vi "Control Limelight.vi"(0 "Read Data Loop Time (ms) (min 10)":u32, 2 "Write Data Loop Time (ms)":u32) -> ()   [LabVIEW 2018]
uses:
  <vilib>/Rock Robotics/Network Tables/NT Read Number.vi
  Robot Global Data.vi
  <vilib>/Rock Robotics/Network Tables/NT Write Number.vi
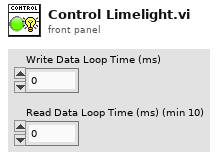
[diagram p1: front panel]
types:
  T1 = cluster{"offsetAngle H":dbl, "offsetAngle V":dbl, "area":dbl, "skew":dbl, "validTarget":dbl, "latency":dbl}
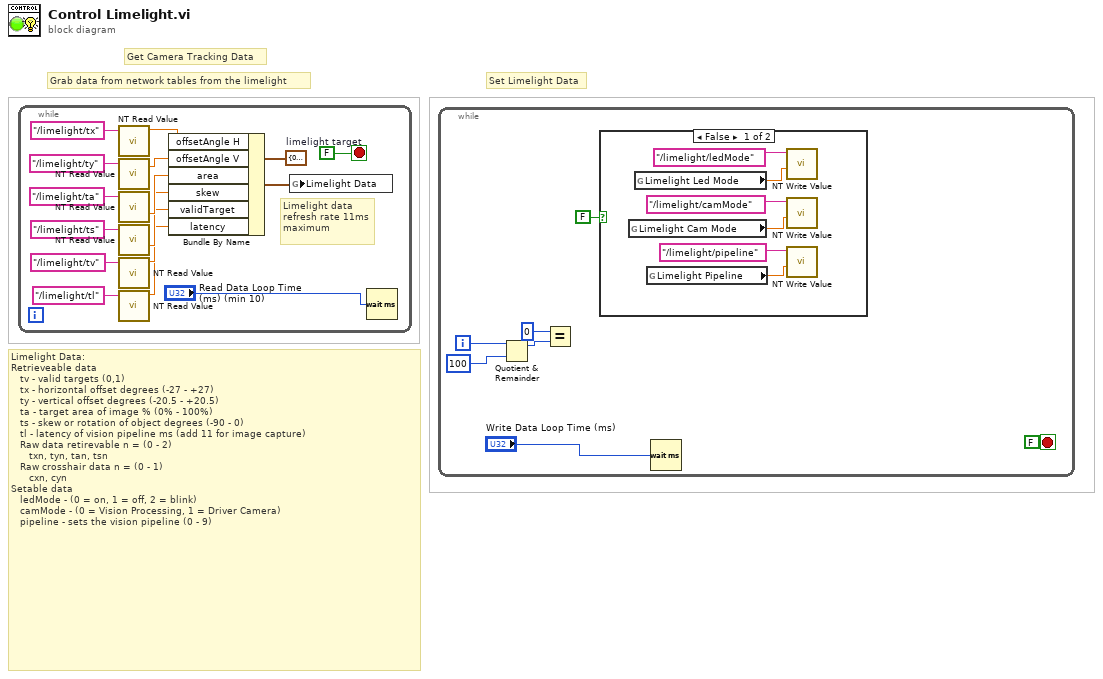
[diagram p0: block diagram]
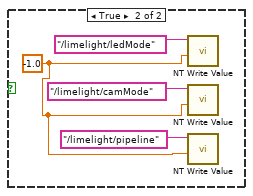
[diagram p2: hidden frame]
diagram:
  # "Set Limelight Data"
  # "Limelight Data:\nRetrieveable data\n   tv - valid targets (0,1)\n   tx - horizontal offset degrees (-27 - +27)\n   ty - vertical offset degrees (-20.5 - +20.5)\n   ta - target area of image % (0% - 100%)\n   ts - skew or rotation of object degrees (-90 - 0)\n   tl - latency of vision pipeline ms (add 11 for image capture)\n   Raw data retirevable n = (0 - 2)\n      txn, tyn, tan, tsn\n   Raw crosshair data n = (0 - 1)\n      cxn, cyn\nSetable data\n   ledMode - (0 = on, 1 = off, 2 = blink)\n   camMode - (0 = Vision Processing, 1 = Driver Camera)\n   pipeline - sets the vision pipeline (0 - 9)"
  # "Grab data from network tables from the limelight"
  # "Get Camera Tracking Data"
  n1 = while {
    stop <- FALSE stop-if-true
    w12 = T1 {"offsetAngle H"=0.0, "offsetAngle V"=0.0, "area"=0.0, "skew"=0.0, "validTarget"=0.0, "latency"=0.0}  # limelight target
    # "Limelight data\nrefresh rate 11ms\nmaximum"
    n2 = call-poly <vilib>:"NT Read Value.vi"("Name"="/limelight/tx") -> ("Numeric"=w11:dbl)  [unwired: 9 in, 1 out]
    n3 = call-poly <vilib>:"NT Read Value.vi"("Name"="/limelight/ty") -> ("Numeric"=w10:dbl)  [unwired: 9 in, 1 out]
    n4 = call-poly <vilib>:"NT Read Value.vi"("Name"="/limelight/ta") -> ("Numeric"=w9:dbl)  [unwired: 9 in, 1 out]
    n5 = call-poly <vilib>:"NT Read Value.vi"("Name"="/limelight/ts") -> ("Numeric"=w8:dbl)  [unwired: 9 in, 1 out]
    n6 = call-poly <vilib>:"NT Read Value.vi"("Name"="/limelight/tv") -> ("Numeric"=w4:dbl)  [unwired: 9 in, 1 out]
    n7 = call-poly <vilib>:"NT Read Value.vi"("Name"="/limelight/tl") -> ("Numeric"=w2:dbl)  [unwired: 9 in, 1 out]
    n8 = Bundle By Name(cluster=w12, "offsetAngle H"=w11, "offsetAngle V"=w10, "area"=w9, "skew"=w8, "validTarget"=w4, "latency"=w2) -> (w6:T1)
    n9 = global write "Robot Global Data.vi" "Limelight Data"(w6) -> ()
    n10 = Wait (ms)(milliseconds to wait="Read Data Loop Time (ms) (min 10)") -> ()  [unwired: 1 out]
  }
  n11 = while {
    i -> [w21]
    stop <- FALSE stop-if-true
    n12 = Quotient & Remainder(x=w21, y=100) -> (x-y*floor(x/y)=w19:i32)  [unwired: 1 out]
    n13 = Equal?(x=0, y=w19) -> ()  [unwired: 1 out]
    n14 = case shown="False" FALSE {
      frame False {
        n15 = global read "Robot Global Data.vi" "Limelight Cam Mode"() -> (w25:dbl)
        n16 = global read "Robot Global Data.vi" "Limelight Led Mode"() -> (w26:dbl)
        n17 = global read "Robot Global Data.vi" "Limelight Pipeline"() -> (w24:dbl)
        n18 = call-poly <vilib>:"NT Write Value.vi"("Numeric"=w26, "Name"="/limelight/ledMode") -> ()  [unwired: 9 in, 1 out]
        n19 = call-poly <vilib>:"NT Write Value.vi"("Numeric"=w25, "Name"="/limelight/camMode") -> ()  [unwired: 9 in, 1 out]
        n20 = call-poly <vilib>:"NT Write Value.vi"("Numeric"=w24, "Name"="/limelight/pipeline") -> ()  [unwired: 9 in, 1 out]
      }
      frame True {
        w30 = -1.0
        n21 = call-poly <vilib>:"NT Write Value.vi"("Numeric"=w30, "Name"="/limelight/ledMode") -> ()  [unwired: 9 in, 1 out]
        n22 = call-poly <vilib>:"NT Write Value.vi"("Numeric"=w30, "Name"="/limelight/camMode") -> ()  [unwired: 9 in, 1 out]
        n23 = call-poly <vilib>:"NT Write Value.vi"("Numeric"=w30, "Name"="/limelight/pipeline") -> ()  [unwired: 9 in, 1 out]
      }
    }
    n24 = Wait (ms)(milliseconds to wait="Write Data Loop Time (ms)") -> ()  [unwired: 1 out]
  }
